vi "PL Measure.vi"() -> ()   [LabVIEW 2017]
uses:
  Program Files (x86)/National Instruments/LabVIEW 2014/instr.lib/Keithley 2600 Series/Public/Channel.ctl
  Program Files (x86)/National Instruments/LabVIEW 2014/instr.lib/Keithley 2600 Series/Keithley 2600 Series.lvlib
panel:
  out "Time":dbl[](array[numeric]) format="%^#_6e"
  out "error out":errorcluster
  out "Current":dbl[](array[numeric]) format="%^#_6e"
  in  "Run":bool
  in  "NPLC":dbl format="%#_13g"
  in  "Background Time (s)":dbl format="%#_13g"
  in  "Interval (ms)":dbl format="%#_13g"
  in  "Time (s)":dbl format="%#_13g"
  in  "error in (no error)":errorcluster
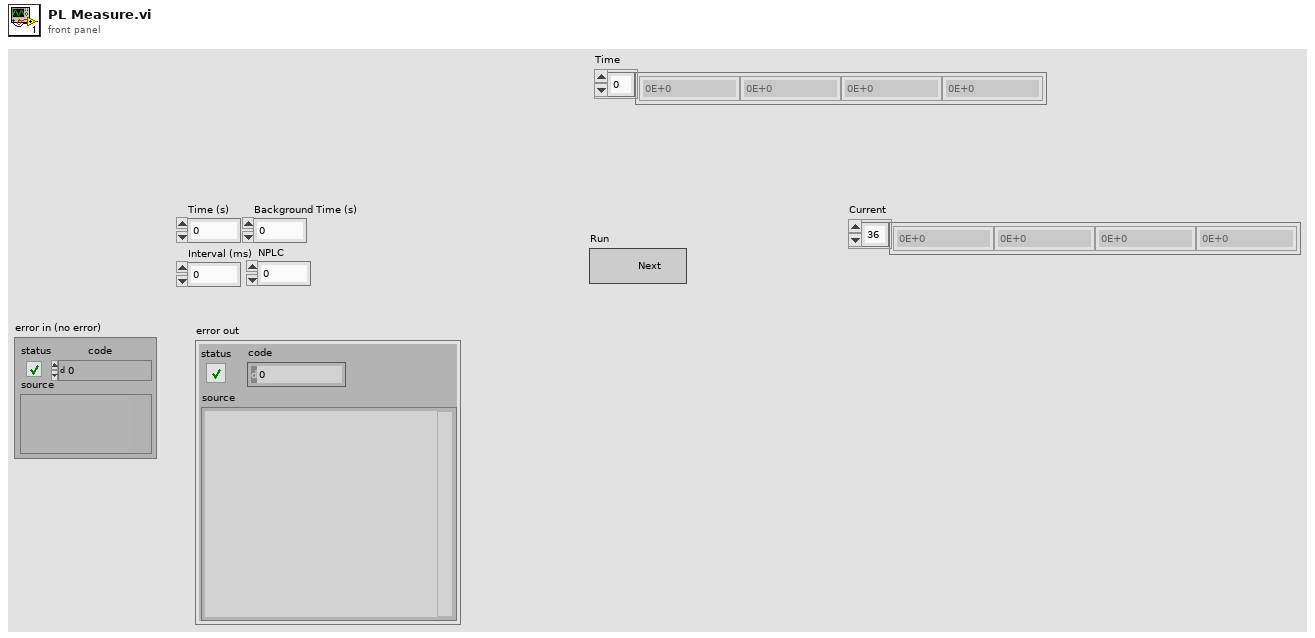
[diagram p1: front panel]
types:
  T1 = enum32{"Normal", "Big Endian", "Little Endian", "Network", "Swapped"}
  T2 = enum32{"ASCII", "Real 32", "Real 64", "Single Precision Real", "Double Precision Real"}
  T3 = typedef "Keithley 2600 Series.lvlib/Channel.ctl" = enum32{"Channel A", "Channel B"}
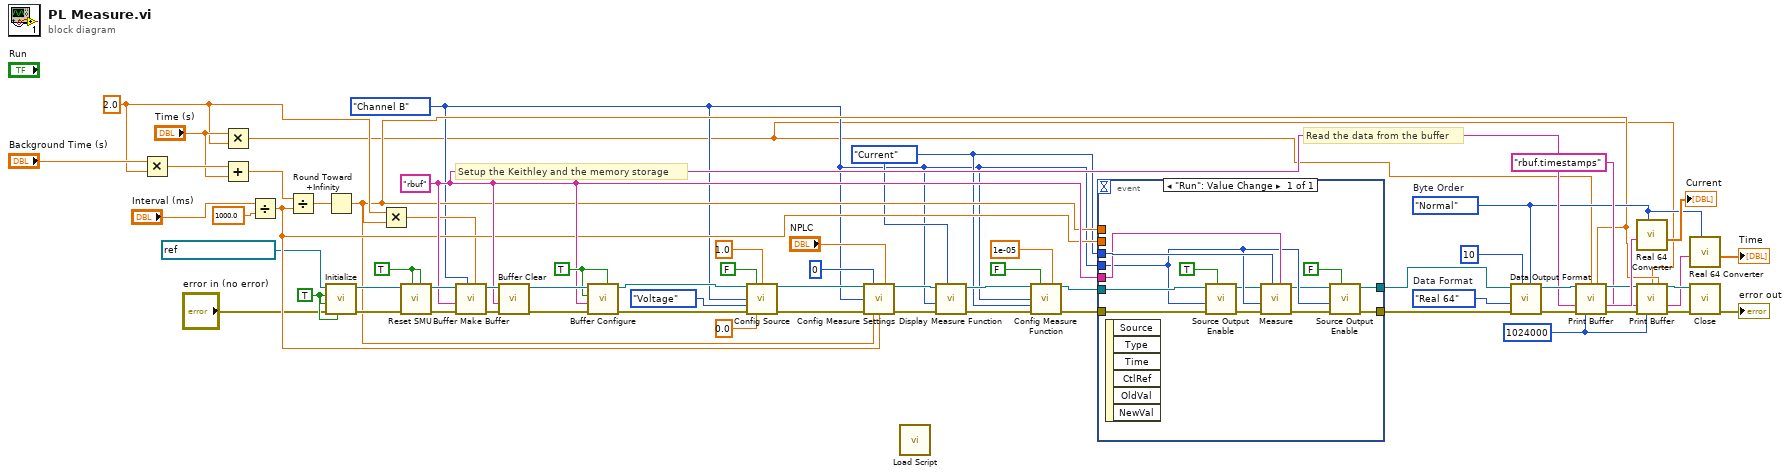
[diagram p0: block diagram]
diagram:
  w20 = T1."Normal"  # Byte Order
  w23 = u32 1024000 ("Byte Count (1024)")
  w36 = T2."Real 64"  # Data Format
  w5 = enum32{"Current", "Voltage"}."Current" ("Function (Current)")
  w12 = 2.0
  w51 = TRUE
  w4 = Channel."Channel B" ("x")
  w57 = TRUE
  w58 = TRUE
  w31 = "rbuf"
  # "Read the data from the buffer"
  # "Setup the Keithley and the memory storage"
  n1 = Multiply(x="Background Time (s)", y=w12) -> (x*y=w44:dbl)
  n2 = Multiply(x="Time (s)", y=w12) -> (x*y=w3:dbl)
  n3 = Add(x=w44, y="Time (s)") -> (x+y=w43:dbl)
  n4 = Divide(x="Interval (ms)", y=1000.0) -> (x/y=w15:dbl)
  n5 = Divide(x=w43, y=w15) -> (x/y=w42:dbl)
  n6 = Round Toward +Infinity(x=w42) -> (ceil(x): smallest int >= x=w11:dbl)
  n7 = call "Initialize.vi"("Reset (True)"=w57, "error in (no error)"="error in (no error)", "Error Query (False)"=w57, "ID Query (True)"=w57, "VISA resource name"=refnum<visa-resource-name> "GPIB0::26::INSTR") -> ("error out"=w55:errorcluster, "VISA resource name out"=w56:refnum<visa-resource-name>)  [unwired: 5 in]
  n8 = Multiply(x=w12, y=w11) -> (x*y=w10:dbl)
  n9 = call "Reset SMU.vi"("SMU B (No)"=w51, "SMU A (No)"=w51, "error in (no error)"=w55, "VISA resource name"=w56) -> ("error out"=w63:errorcluster, "VISA resource name out"=w64:refnum<visa-resource-name>)  [unwired: 4 in, 2 out]
  n10 = call "Buffer Make Buffer.vi"("Capacity (1)"=w10, "Channel (Channel A)"=w4, "error in (no error)"=w63, "Buffer Name (buf)"=w31, "VISA resource name"=w64) -> ("error out"=w61:errorcluster, "VISA resource name out"=w62:refnum<visa-resource-name>)  [unwired: 3 in, 2 out]
  n11 = call "Buffer Clear.vi"("error in (no error)"=w61, "Buffer Name"=w31, "VISA resource name"=w62) -> ("error out"=w59:errorcluster, "VISA resource name out"=w60:refnum<visa-resource-name>)  [unwired: 6 in, 1 out]
  n12 = call "Buffer Configure.vi"("Collect Timestamps (Off)"=w58, "error in (no error)"=w59, "Buffer Name"=w31, "Append Mode (Off)"=w58, "VISA resource name"=w60) -> ("error out"=w54:errorcluster, "VISA resource name out"=w49:refnum<visa-resource-name>)  [unwired: 4 in, 1 out]
  n13 = call "Config Source.vi"("VISA resource name"=w49, "Autorange (On)"=FALSE, "Range (1.000)"=1.0, "Channel (Channel A)"=w4, "Function (Current)"=enum32{"Current", "Voltage"}."Voltage", "error in"=w54, "Level (0.000)"=0.0) -> ("VISA resource name out"=w47:refnum<visa-resource-name>, "error out"=w46:errorcluster)  [unwired: 4 in, 3 out]
  n14 = call "Config Measure Settings.vi"("VISA resource name"=w47, "Autozero (Auto)"=0, "NPLC (1.000)"="NPLC", "Channel (Channel A)"=w4, "error in"=w46, "Measure Count (1)"=w11, "Interval (0.000)"=w15) -> ("VISA resource name out"=w8:refnum<visa-resource-name>, "error out"=w9:errorcluster)  [unwired: 5 in, 2 out]
  n15 = call "Load Script.vi"() -> ()  [unwired: 9 in, 3 out]
  n16 = call "Display Measure Function.vi"("Function (Current)"=w5, "error in (no error)"=w9, "Channel (Channel A)"=w4, "VISA resource name"=w8) -> ("error out"=w6:errorcluster, "VISA resource name out"=w7:refnum<visa-resource-name>)  [unwired: 4 in, 2 out]
  n17 = call "Config Measure Function.vi"("VISA resource name"=w7, "Autorange (On)"=FALSE, "Range (1.000)"=1e-05, "Channel (Channel A)"=w4, "Function (Current)"=w5, "error in"=w6) -> ("VISA resource name out"=w40:refnum<visa-resource-name>, "error out"=w39:errorcluster)  [unwired: 6 in, 2 out]
  n18 = event shown="[0] \"Run\": Value Change" {
    selector: _ -> [_]
    dyn-events: _ -> [_]
    timeout: _ -> [_]
    tunnel: w40 -> [w77]
    tunnel: w39 -> [w76]
    tunnel: w4 -> [w72]
    tunnel: w5 -> [w74]
    tunnel: w31 -> [w73]
    tunnel: [w67] -> w34
    tunnel: [w68] -> w33
    tunnel: w11 -> [_]
    tunnel: w15 -> [_]
    event "Run": Value Change {
      n19 = event-data() -> ()  [unwired: 1 in, 6 out]
      n20 = call "Source Output Enable.vi"("Output (Off)"=TRUE, "error in (no error)"=w76, "Channel (Channel A)"=w72, "VISA resource name"=w77) -> ("error out"=w65:errorcluster, "VISA resource name out"=w66:refnum<visa-resource-name>)  [unwired: 4 in, 2 out]
      n21 = call "Measure.vi"("Buffer 1"=w73, "Function (Current)"=w74, "error in (no error)"=w65, "Channel (Channel A)"=w72, "VISA resource name"=w66) -> ("error out"=w71:errorcluster, "VISA resource name out"=w70:refnum<visa-resource-name>)  [unwired: 2 in, 3 out]
      n22 = call "Source Output Enable.vi"("Output (Off)"=FALSE, "error in (no error)"=w71, "Channel (Channel A)"=w72, "VISA resource name"=w70) -> ("error out"=w67:errorcluster, "VISA resource name out"=w68:refnum<visa-resource-name>)  [unwired: 4 in, 2 out]
    }
  }
  n23 = call "Data Output Format.vi"("Byte Order (Normal)"=w20, "ASCII Precision (6)"=10, "error in (no error)"=w34, "Data Format (ASCII)"=w36, "VISA resource name"=w33) -> ("error out"=w37:errorcluster, "VISA resource name out"=w38:refnum<visa-resource-name>)  [unwired: 1 in, 4 out]
  n24 = call "Print Buffer.vi"("VISA resource name"=w38, "Timeout (2000 ms)"=w3, "End Index (1)"=w11, "Buffer Name(s)"=w31, "error in (no error)"=w37, "Byte Count (1024)"=w23) -> ("VISA resource name out"=w25:refnum<visa-resource-name>, "Buffer Data"=w35:string, "error out"=w24:errorcluster)  [unwired: 1 in, 6 out]
  n25 = call "Real 64 Converter.vi"("Byte Order (Normal)"=w20, "Data In"=w35) -> ("Data Array Out"=→"Current":dbl[])  [unwired: 9 in]
  n26 = call "Print Buffer.vi"("VISA resource name"=w25, "Timeout (2000 ms)"=w3, "End Index (1)"=w11, "Buffer Name(s)"="rbuf.timestamps", "error in (no error)"=w24, "Byte Count (1024)"=w23) -> ("VISA resource name out"=w27:refnum<visa-resource-name>, "Buffer Data"=w21:string, "error out"=w26:errorcluster)  [unwired: 1 in, 6 out]
  n27 = call "Real 64 Converter.vi"("Byte Order (Normal)"=w20, "Data In"=w21) -> ("Data Array Out"=→"Time":dbl[])  [unwired: 9 in]
  n28 = call "Close.vi"("error in (no error)"=w26, "VISA resource name"=w27) -> ("error out"=→"error out":errorcluster)  [unwired: 9 in]
